vi "fgv_Video Rec Enabled for Live protocols.vi"(9 "Function":T1, 11 "Video Recording Enabled for Live protocols":bool) -> (3 "Video Recording Enabled for Live protocols":bool)   [LabVIEW 2013]
uses:
  Typedefs/Read Write Enum.ctl
panel:
  # "SUBROUTINE"
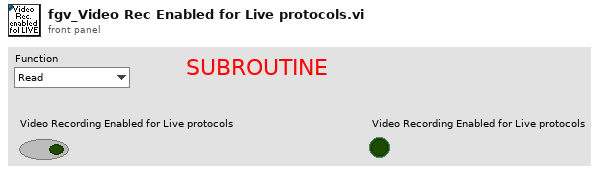
[diagram p1: front panel]
types:
  T1 = typedef "Read Write Enum.ctl" = enum16{"Read", "Write"}
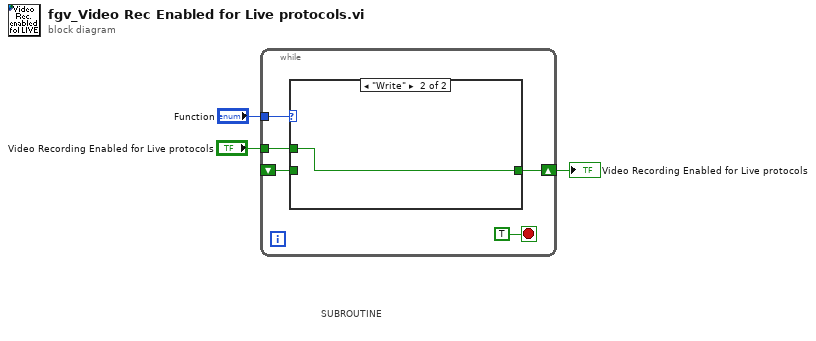
[diagram p0: block diagram]
diagram:
  # "SUBROUTINE"
  n1 = while {
    tunnel: "Function" -> [w7]
    tunnel: "Video Recording Enabled for Live protocols" -> [w6]
    shift-right: [w5] -> w1
    shift-left: _ -> [w4]
    stop <- TRUE stop-if-true
    n2 = case shown="\"Write\"" w7 {
      tunnel: w6 -> [_ w10]
      tunnel: [w9 w10] -> w5
      tunnel: w4 -> [w9 _]
      frame "Read", Default {
      }
      frame "Write" {
      }
    }
  }
  "Video Recording Enabled for Live protocols" <- w1
